vi "Read VISA resource name.vi"(8 "error in (no error)":errorcluster, 11 "Abstract Camera in":refnum<class "Abstract Camera.lvclass">) -> (0 "error out":errorcluster, 2 "VISA resource name":refnum<visa-resource-name>, 3 "Abstract Camera out":refnum<class "Abstract Camera.lvclass">)   [LabVIEW 2019, in "Abstract Camera.lvclass"]
uses:
  Abstract Camera.lvclass
  Abstract Camera.lvclass/Abstract Camera.ctl
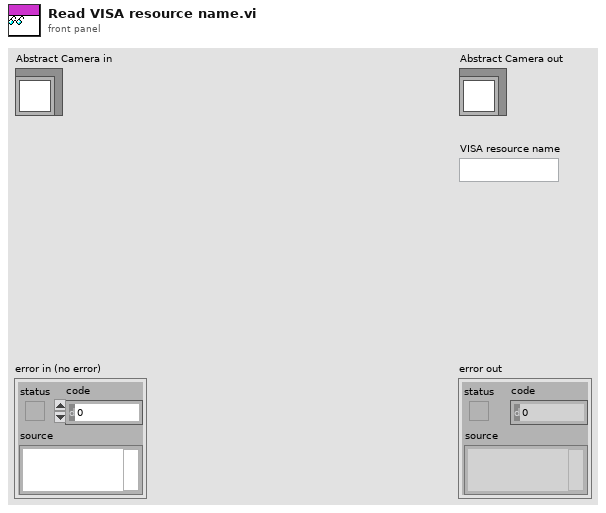
[diagram p1: front panel]
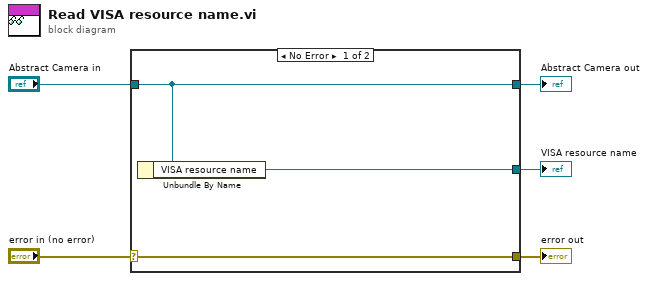
[diagram p0: block diagram]
diagram:
  n1 = case shown="No Error" "error in (no error)" {
    selector: "error in (no error)" -> [w8 w9]
    tunnel: [w8 w9] -> w4
    tunnel: [w7 w10] -> w2
    tunnel: "Abstract Camera in" -> [w7 w10]
    tunnel: [w6 _] -> w1
    frame No Error {
      n2 = Unbundle By Name(w7) -> ("VISA resource name"=w6:refnum<visa-resource-name>)
    }
    frame Error {
    }
  }
  "error out" <- w4
  "Abstract Camera out" <- w2
  "VISA resource name" <- w1
